vi "16-QAM_Constellation.vi"() -> ()   [LabVIEW 2014]
uses:
  <vilib>/Analysis/NI_AALBase.lvlib
panel:
  out "x/y 2":dbl
  out "x/y":dbl
  out "XY Graph 2":cluster{dbl[], dbl[]}(graph)
  in  "standard deviation":dbl=1.0000000000000002 format="%0.2f"
  out "XY Graph":cdb[](graph)
  out "Array":i32[](array[numeric])
  in  "Numeric":i32
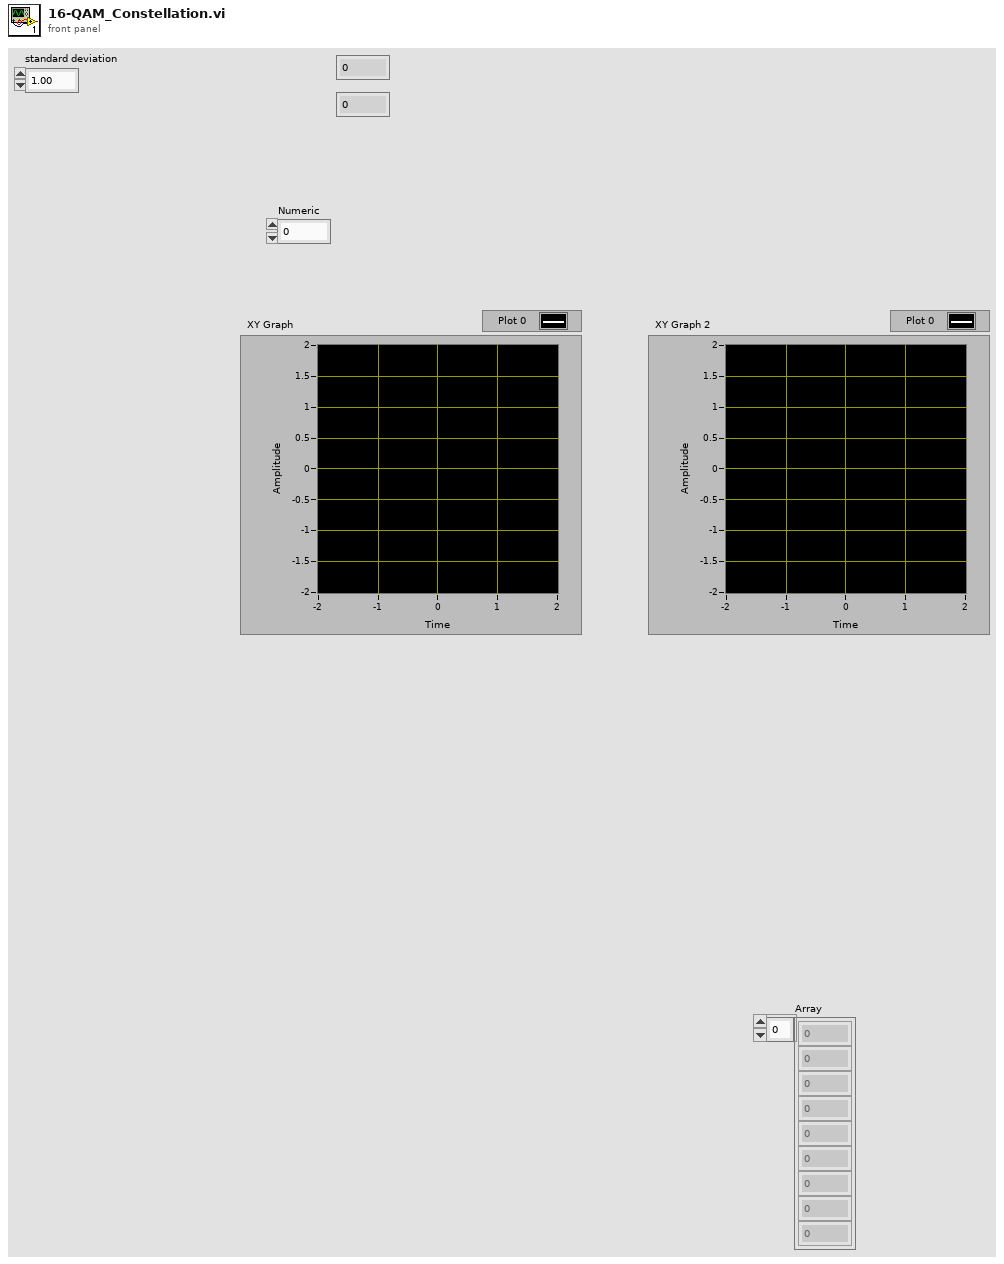
[diagram p1: front panel]
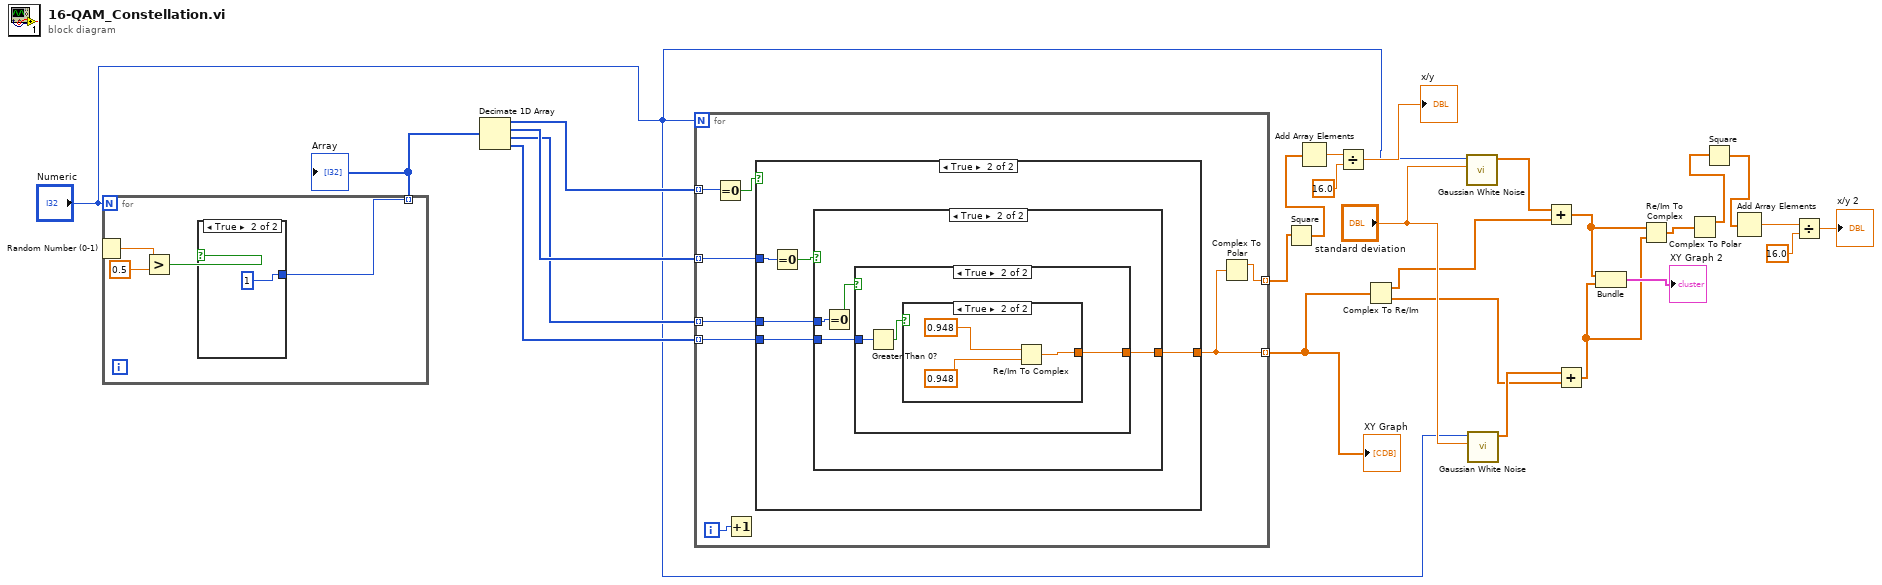
[diagram p0: block diagram]
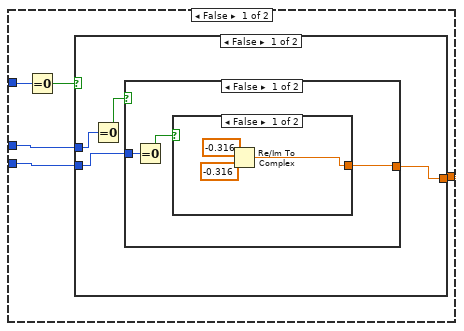
[diagram p2: hidden frame]
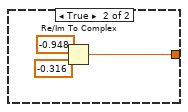
[diagram p3: hidden frame]
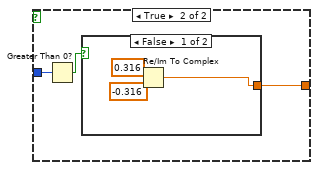
[diagram p4: hidden frame]
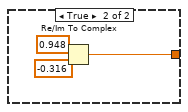
[diagram p5: hidden frame]
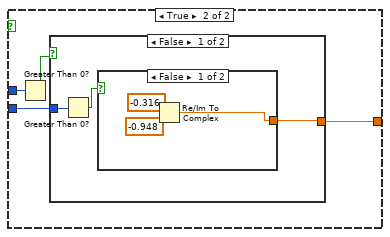
[diagram p6: hidden frame]
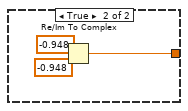
[diagram p7: hidden frame]
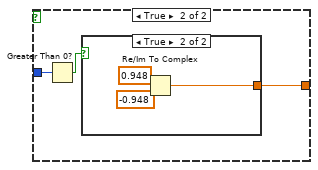
[diagram p8: hidden frame]
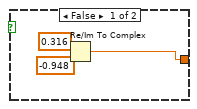
[diagram p9: hidden frame]
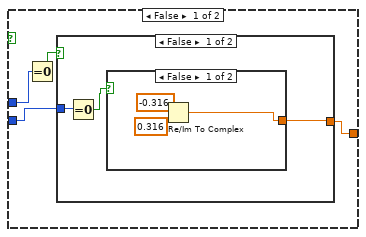
[diagram p10: hidden frame]
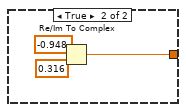
[diagram p11: hidden frame]
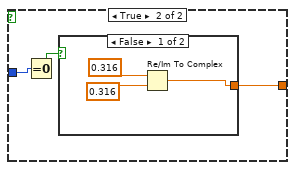
[diagram p12: hidden frame]
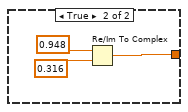
[diagram p13: hidden frame]
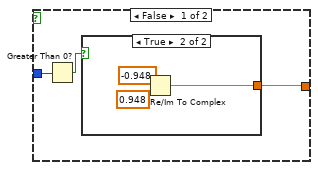
[diagram p14: hidden frame]
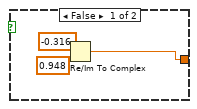
[diagram p15: hidden frame]
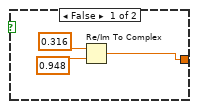
[diagram p16: hidden frame]
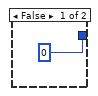
[diagram p17: hidden frame]
diagram:
  n1 = for {
    N: "Numeric" -> [_]
    tunnel: [w28] -> w26 mode=indexing
    n2 = Random Number (0-1)() -> (number: 0 to 1=w29:dbl)
    n3 = Greater?(x=w29, y=0.5) -> (0:w27:bool)
    n4 = case shown="True" w27 {
      tunnel: [0 1] -> w28
      frame False {
      }
      frame True {
      }
    }
  }
  "Array" <- w26
  n5 = Decimate 1D Array(w26) -> (w25:i32[], w24:i32[], w23:i32[], w22:i32[])
  n6 = for {
    N: "Numeric" -> [_]
    tunnel: w25 -> [w37] mode=indexing
    tunnel: w24 -> [w40] mode=indexing
    tunnel: w23 -> [w39] mode=indexing
    tunnel: w22 -> [w38] mode=indexing
    tunnel: [w35] -> w21 mode=indexing
    tunnel: [w34] -> w4 mode=indexing
    i -> [w33]
    n7 = Equal To 0?(x=w37) -> (x = 0?=w36:bool)
    n8 = Increment(x=w33) -> ()  [unwired: 1 out]
    n9 = case shown="True" w36 {
      tunnel: w40 -> [w41 w90]
      tunnel: w39 -> [w45 w94]
      tunnel: w38 -> [w44 w93]
      tunnel: [w43 w92] -> w35
      frame False {
        n10 = Equal To 0?(x=w41) -> (x = 0?=w42:bool)
        n11 = case shown="False" w42 {
          tunnel: w45 -> [w46 w71]
          tunnel: w44 -> [w49 w70]
          tunnel: [w48 w68] -> w43
          frame False {
            n12 = Equal To 0?(x=w46) -> (x = 0?=w47:bool)
            n13 = case shown="False" w47 {
              tunnel: w49 -> [w50 w61]
              tunnel: [w52 w59] -> w48
              frame False {
                n14 = Equal To 0?(x=w50) -> (x = 0?=w51:bool)
                n15 = case shown="False" w51 {
                  tunnel: [w53 w58] -> w52
                  frame False {
                    n16 = Re/Im To Complex(1:-0.316, 2:-0.316) -> (0:w53:cdb)
                  }
                  frame True {
                    n17 = Re/Im To Complex(1:-0.316, 2:-0.948) -> (0:w58:cdb)
                  }
                }
              }
              frame True {
                n18 = Greater Than 0?(x=w61) -> (x > 0?=w60:bool)
                n19 = case shown="False" w60 {
                  tunnel: [w62 w67] -> w59
                  frame False {
                    n20 = Re/Im To Complex(1:-0.316, 2:0.316) -> (0:w62:cdb)
                  }
                  frame True {
                    n21 = Re/Im To Complex(1:-0.316, 2:0.948) -> (0:w67:cdb)
                  }
                }
              }
            }
          }
          frame True {
            n22 = Greater Than 0?(x=w71) -> (x > 0?=w69:bool)
            n23 = case shown="False" w69 {
              tunnel: w70 -> [w72 w83]
              tunnel: [w73 w81] -> w68
              frame False {
                n24 = Greater Than 0?(x=w72) -> (x > 0?=w74:bool)
                n25 = case shown="False" w74 {
                  tunnel: [w75 w80] -> w73
                  frame False {
                    n26 = Re/Im To Complex(1:-0.948, 2:-0.316) -> (0:w75:cdb)
                  }
                  frame True {
                    n27 = Re/Im To Complex(1:-0.948, 2:-0.948) -> (0:w80:cdb)
                  }
                }
              }
              frame True {
                n28 = Greater Than 0?(x=w83) -> (x > 0?=w82:bool)
                n29 = case shown="True" w82 {
                  tunnel: [w84 w89] -> w81
                  frame False {
                    n30 = Re/Im To Complex(1:-0.948, 2:0.316) -> (0:w84:cdb)
                  }
                  frame True {
                    n31 = Re/Im To Complex(1:-0.948, 2:0.948) -> (0:w89:cdb)
                  }
                }
              }
            }
          }
        }
      }
      frame True {
        n32 = Equal To 0?(x=w90) -> (x = 0?=w91:bool)
        n33 = case shown="True" w91 {
          tunnel: w94 -> [w95 w117]
          tunnel: w93 -> [w98 w120]
          tunnel: [w97 w119] -> w92
          frame False {
            n34 = Equal To 0?(x=w95) -> (x = 0?=w96:bool)
            n35 = case shown="False" w96 {
              tunnel: w98 -> [w99 w108]
              tunnel: [w101 w110] -> w97
              frame False {
                n36 = Equal To 0?(x=w99) -> (x = 0?=w100:bool)
                n37 = case shown="False" w100 {
                  tunnel: [w102 w107] -> w101
                  frame False {
                    n38 = Re/Im To Complex(1:0.316, 2:-0.316) -> (0:w102:cdb)
                  }
                  frame True {
                    n39 = Re/Im To Complex(1:0.316, 2:-0.948) -> (0:w107:cdb)
                  }
                }
              }
              frame True {
                n40 = Equal To 0?(x=w108) -> (x = 0?=w109:bool)
                n41 = case shown="False" w109 {
                  tunnel: [w111 w116] -> w110
                  frame False {
                    n42 = Re/Im To Complex(1:0.316, 2:0.316) -> (0:w111:cdb)
                  }
                  frame True {
                    n43 = Re/Im To Complex(1:0.316, 2:0.948) -> (0:w116:cdb)
                  }
                }
              }
            }
          }
          frame True {
            n44 = Equal To 0?(x=w117) -> (x = 0?=w118:bool)
            n45 = case shown="True" w118 {
              tunnel: w120 -> [w121 w132]
              tunnel: [w122 w130] -> w119
              frame False {
                n46 = Greater Than 0?(x=w121) -> (x > 0?=w123:bool)
                n47 = case shown="True" w123 {
                  tunnel: [w124 w129] -> w122
                  frame False {
                    n48 = Re/Im To Complex(1:0.948, 2:-0.316) -> (0:w124:cdb)
                  }
                  frame True {
                    n49 = Re/Im To Complex(1:0.948, 2:-0.948) -> (0:w129:cdb)
                  }
                }
              }
              frame True {
                n50 = Greater Than 0?(x=w132) -> (x > 0?=w131:bool)
                n51 = case shown="True" w131 {
                  tunnel: [w133 w138] -> w130
                  frame False {
                    n52 = Re/Im To Complex(1:0.948, 2:0.316) -> (0:w133:cdb)
                  }
                  frame True {
                    n53 = Re/Im To Complex(1:0.948, 2:0.948) -> (0:w138:cdb)
                  }
                }
              }
            }
          }
        }
      }
    }
    n54 = Complex To Polar(r * e^(i*theta)=w35) -> (r=w34:dbl)  [unwired: 1 out]
  }
  "XY Graph" <- w21
  n55 = Square(x=w4) -> (x^2=w5:dbl[])
  n56 = Add Array Elements(numeric array=w5) -> (sum=w11:dbl)
  n57 = Divide(x=w11, y=16.0) -> (x/y=→"x/y":dbl)
  n58 = Complex To Re/Im(x + iy=w21) -> (x=w18:dbl[], y=w16:dbl[])
  n59 = call <vilib>:"Gaussian White Noise.vi"("standard deviation"="standard deviation", "samples"="Numeric") -> ("Gaussian noise pattern"=w19:dbl[])  [unwired: 8 in, 1 out]
  n60 = call <vilib>:"Gaussian White Noise.vi"("standard deviation"="standard deviation", "samples"="Numeric") -> ("Gaussian noise pattern"=w17:dbl[])  [unwired: 8 in, 1 out]
  n61 = Add(x=w19, y=w18) -> (x+y=w14:dbl[])
  n62 = Add(x=w17, y=w16) -> (x+y=w13:dbl[])
  n63 = Bundle(w14, w13) -> (→"XY Graph 2":cluster{dbl[], dbl[]})  [unwired: 1 in]
  n64 = Re/Im To Complex(1:w13, 2:w14) -> (0:w12:cdb[])
  n65 = Complex To Polar(r * e^(i*theta)=w12) -> (r=w3:dbl[])  [unwired: 1 out]
  n66 = Square(x=w3) -> (x^2=w2:dbl[])
  n67 = Add Array Elements(numeric array=w2) -> (sum=w8:dbl)
  n68 = Divide(x=w8, y=16.0) -> (x/y=→"x/y 2":dbl)
